vi "Canwrite_jetson.vi"(10 "클러스터":T1={"L_velocity"=0, "L_angle"=0.0, "L_Peak start"=10.0, "L_Release start"=36.0, "R_velocity"=0, "R_angle"=0.0, "R_Peak start"=10.0, "R_Release start"=36.0}) -> (2 "배열":T2(array[cluster]))   [LabVIEW 2019]
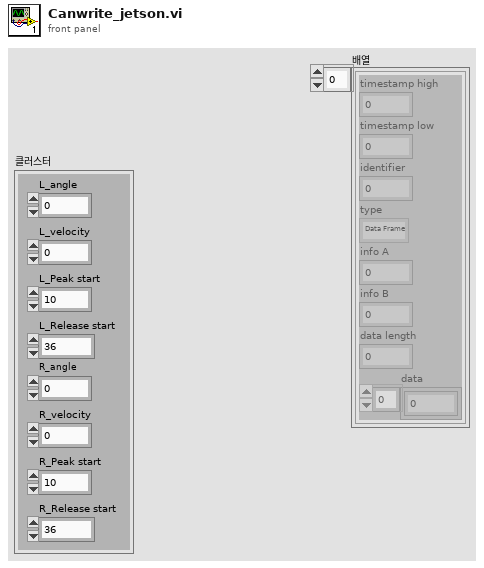
[diagram p1: front panel]
types:
  T1 = cluster{"L_velocity":u32, "L_angle":sgl, "L_Peak start":sgl, "L_Release start":sgl, "R_velocity":u32, "R_angle":sgl, "R_Peak start":sgl, "R_Release start":sgl}
  T2 = cluster{"timestamp high":u32, "timestamp low":u32, "identifier":u32, "type":enum8{"Data Frame", "Remote Frame", "(reserved)", "(reserved) ", "(reserved)  ", "(reserved)   ", "Bus Error", "Transceiver Fault"}, "info A":u8, "info B":u8, "data length":u8, "data":u8[]}[]
  T3 = enum8{"Data Frame", "Remote Frame", "(reserved)", "(reserved) ", "(reserved)  ", "(reserved)   ", "Bus Error", "Transceiver Fault"}
  T4 = cluster{"timestamp high":u32, "timestamp low":u32, "identifier":u32, "type":enum8{"Data Frame", "Remote Frame", "(reserved)", "(reserved) ", "(reserved)  ", "(reserved)   ", "Bus Error", "Transceiver Fault"}, "info A":u8, "info B":u8, "data length":u8, "data":u8[]}
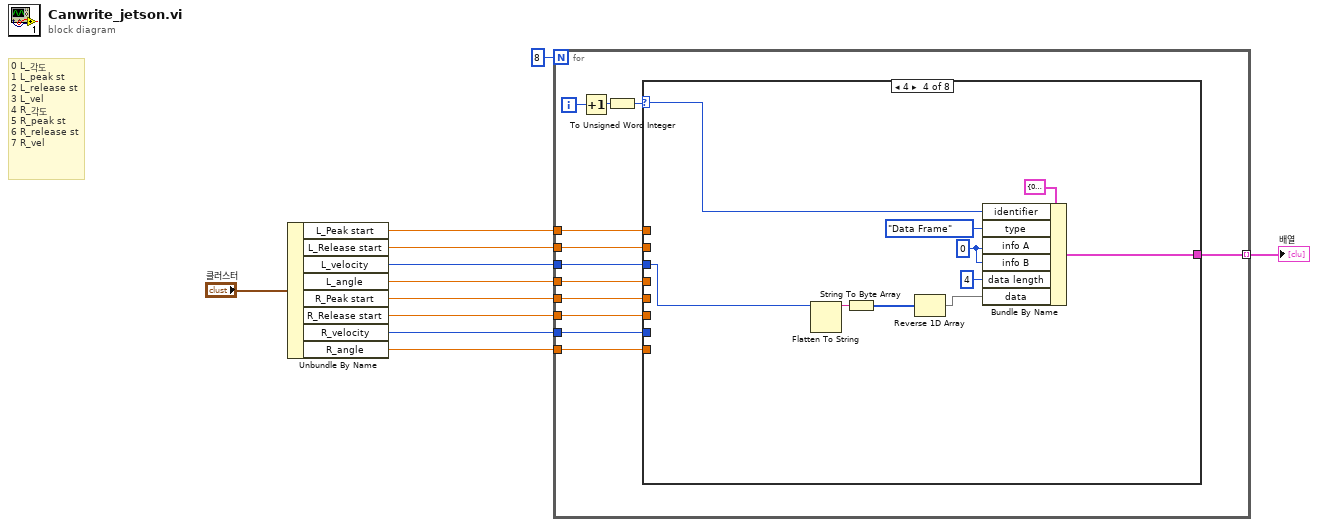
[diagram p0: block diagram]
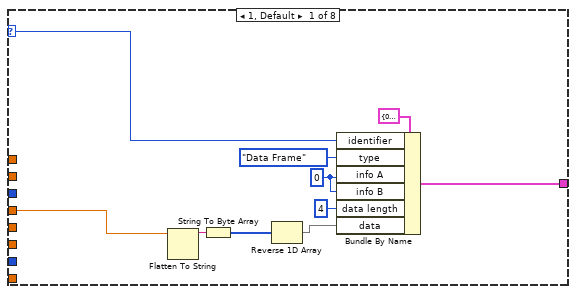
[diagram p2: hidden frame]
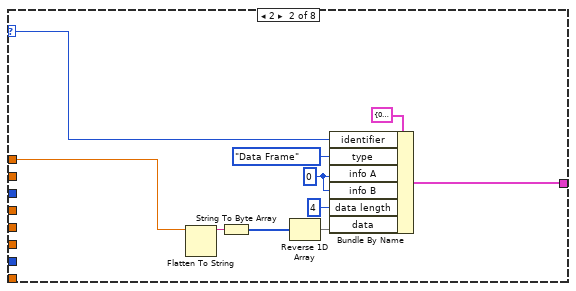
[diagram p3: hidden frame]
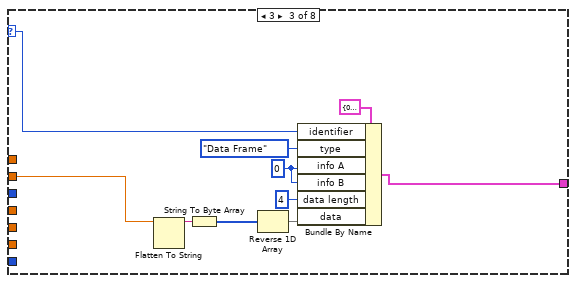
[diagram p4: hidden frame]
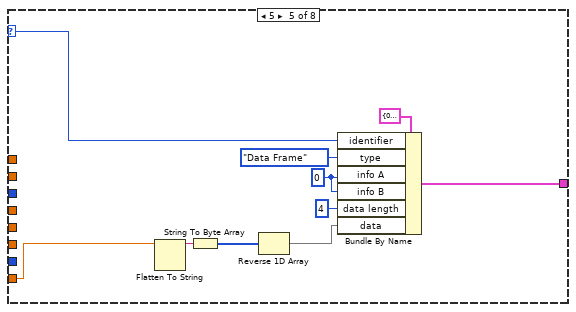
[diagram p5: hidden frame]
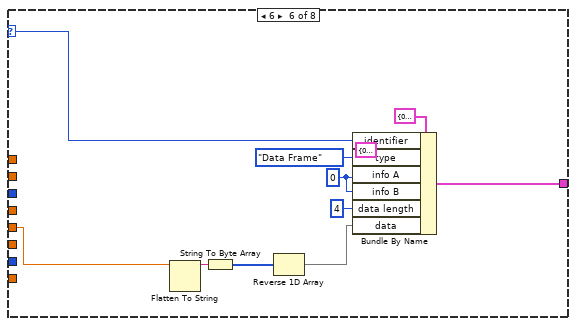
[diagram p6: hidden frame]
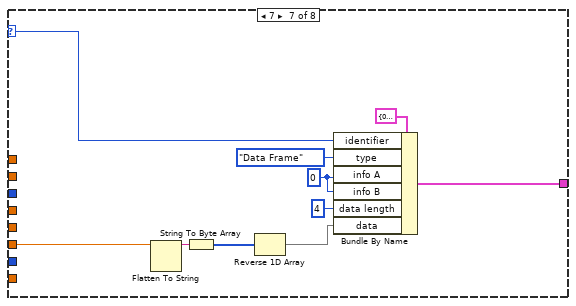
[diagram p7: hidden frame]
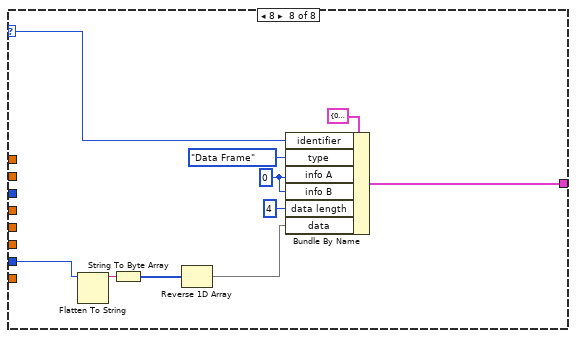
[diagram p8: hidden frame]
diagram:
  # "0 L_각도\n1 L_peak st\n2 L_release st\n3 L_vel\n4 R_각도\n5 R_peak st\n6 R_release st\n7 R_vel"
  n1 = Unbundle By Name("클러스터") -> ("L_Peak start"=w8:sgl, "L_Release start"=w6:sgl, "L_velocity"=w7:u32, "L_angle"=w5:sgl, "R_Peak start"=w4:sgl, "R_Release start"=w3:sgl, "R_velocity"=w2:u32, "R_angle"=w1:sgl)
  n2 = for {
    N: 8 -> [_]
    tunnel: w8 -> [w23]
    tunnel: w6 -> [w22]
    tunnel: w7 -> [w20]
    tunnel: [w21] -> w10 mode=indexing
    tunnel: w5 -> [w16]
    tunnel: w4 -> [w15]
    tunnel: w3 -> [w14]
    tunnel: w2 -> [w13]
    tunnel: w1 -> [w12]
    i -> [w19]
    n3 = Increment(x=w19) -> (x+1=w18:i32)
    n4 = To Unsigned Word Integer(number=w18) -> (unsigned 16bit integer=w17:u16)
    n5 = case shown="4" w17 {
      selector: w17 -> [w25 w39 w45 w59 w69 w79 w89 w99]
      tunnel: w23 -> [_ w34 _ _ _ _ _ _]
      tunnel: w22 -> [_ _ w44 _ _ _ _ _]
      tunnel: [w29 w38 w46 w58 w68 w78 w88 w98] -> w21
      tunnel: w20 -> [_ _ _ w54 _ _ _ _]
      tunnel: w16 -> [w24 _ _ _ _ _ _ _]
      tunnel: w15 -> [_ _ _ _ _ w74 _ _]
      tunnel: w14 -> [_ _ _ _ _ _ w84 _]
      tunnel: w13 -> [_ _ _ _ _ _ _ w94]
      tunnel: w12 -> [_ _ _ _ w64 _ _ _]
      frame 1, Default {
        w31 = u8 0 ("info A")
        n6 = Flatten To String(anything=w24) -> (data string=w28:string)  [unwired: 3 in, 2 out]
        n7 = String To Byte Array(string=w28) -> (unsigned byte array=w27:u8[])
        n8 = Reverse 1D Array(array=w27) -> (reversed array=w26:u8[])
        n9 = Bundle By Name(cluster=T4 {"timestamp high"=0, "timestamp low"=0, "identifier"=0, "type"=enum."Data Frame", "info A"=0, "info B"=0, "data length"=0, "data"=[0, 0, 0, 0, 0, 0, 0, 0]} ("출력 클러스터"), "identifier"=w25, "type"=T3."Data Frame", "info A"=w31, "info B"=w31, "data length"=u8 4, "data"=w26) -> (w29:T4)
      }
      frame 2 {
        w41 = u8 0 ("info A")
        n10 = Flatten To String(anything=w34) -> (data string=w37:string)  [unwired: 3 in, 2 out]
        n11 = String To Byte Array(string=w37) -> (unsigned byte array=w36:u8[])
        n12 = Reverse 1D Array(array=w36) -> (reversed array=w35:u8[])
        n13 = Bundle By Name(cluster=T4 {"timestamp high"=0, "timestamp low"=0, "identifier"=0, "type"=enum."Data Frame", "info A"=0, "info B"=0, "data length"=0, "data"=[0, 0, 0, 0, 0, 0, 0, 0]} ("출력 클러스터"), "identifier"=w39, "type"=T3."Data Frame", "info A"=w41, "info B"=w41, "data length"=u8 4, "data"=w35) -> (w38:T4)
      }
      frame 3 {
        w51 = u8 0 ("info A")
        n14 = Flatten To String(anything=w44) -> (data string=w49:string)  [unwired: 3 in, 2 out]
        n15 = String To Byte Array(string=w49) -> (unsigned byte array=w48:u8[])
        n16 = Reverse 1D Array(array=w48) -> (reversed array=w47:u8[])
        n17 = Bundle By Name(cluster=T4 {"timestamp high"=0, "timestamp low"=0, "identifier"=0, "type"=enum."Data Frame", "info A"=0, "info B"=0, "data length"=0, "data"=[0, 0, 0, 0, 0, 0, 0, 0]} ("출력 클러스터"), "identifier"=w45, "type"=T3."Data Frame", "info A"=w51, "info B"=w51, "data length"=u8 4, "data"=w47) -> (w46:T4)
      }
      frame 4 {
        w61 = u8 0 ("info A")
        n18 = Flatten To String(anything=w54) -> (data string=w57:string)  [unwired: 3 in, 2 out]
        n19 = String To Byte Array(string=w57) -> (unsigned byte array=w56:u8[])
        n20 = Reverse 1D Array(array=w56) -> (reversed array=w55:u8[])
        n21 = Bundle By Name(cluster=T4 {"timestamp high"=0, "timestamp low"=0, "identifier"=0, "type"=enum."Data Frame", "info A"=0, "info B"=0, "data length"=0, "data"=[0, 0, 0, 0, 0, 0, 0, 0]} ("출력 클러스터"), "identifier"=w59, "type"=T3."Data Frame", "info A"=w61, "info B"=w61, "data length"=u8 4, "data"=w55) -> (w58:T4)
      }
      frame 5 {
        w71 = u8 0 ("info A")
        n22 = Flatten To String(anything=w64) -> (data string=w67:string)  [unwired: 3 in, 2 out]
        n23 = String To Byte Array(string=w67) -> (unsigned byte array=w66:u8[])
        n24 = Reverse 1D Array(array=w66) -> (reversed array=w65:u8[])
        n25 = Bundle By Name(cluster=T4 {"timestamp high"=0, "timestamp low"=0, "identifier"=0, "type"=enum."Data Frame", "info A"=0, "info B"=0, "data length"=0, "data"=[0, 0, 0, 0, 0, 0, 0, 0]} ("출력 클러스터"), "identifier"=w69, "type"=T3."Data Frame", "info A"=w71, "info B"=w71, "data length"=u8 4, "data"=w65) -> (w68:T4)
      }
      frame 6 {
        (unwired) T4 {"timestamp high"=0, "timestamp low"=0, "identifier"=0, "type"=enum."Data Frame", "info A"=0, "info B"=0, "data length"=0, "data"=[0, 0, 0, 0, 0, 0, 0, 0]} ("출력 클러스터")
        w81 = u8 0 ("info A")
        n26 = Flatten To String(anything=w74) -> (data string=w77:string)  [unwired: 3 in, 2 out]
        n27 = String To Byte Array(string=w77) -> (unsigned byte array=w76:u8[])
        n28 = Reverse 1D Array(array=w76) -> (reversed array=w75:u8[])
        n29 = Bundle By Name(cluster=T4 {"timestamp high"=0, "timestamp low"=0, "identifier"=0, "type"=enum."Data Frame", "info A"=0, "info B"=0, "data length"=0, "data"=[0, 0, 0, 0, 0, 0, 0, 0]} ("출력 클러스터"), "identifier"=w79, "type"=T3."Data Frame", "info A"=w81, "info B"=w81, "data length"=u8 4, "data"=w75) -> (w78:T4)
      }
      frame 7 {
        w91 = u8 0 ("info A")
        n30 = Flatten To String(anything=w84) -> (data string=w87:string)  [unwired: 3 in, 2 out]
        n31 = String To Byte Array(string=w87) -> (unsigned byte array=w86:u8[])
        n32 = Reverse 1D Array(array=w86) -> (reversed array=w85:u8[])
        n33 = Bundle By Name(cluster=T4 {"timestamp high"=0, "timestamp low"=0, "identifier"=0, "type"=enum."Data Frame", "info A"=0, "info B"=0, "data length"=0, "data"=[0, 0, 0, 0, 0, 0, 0, 0]} ("출력 클러스터"), "identifier"=w89, "type"=T3."Data Frame", "info A"=w91, "info B"=w91, "data length"=u8 4, "data"=w85) -> (w88:T4)
      }
      frame 8 {
        w101 = u8 0 ("info A")
        n34 = Flatten To String(anything=w94) -> (data string=w97:string)  [unwired: 3 in, 2 out]
        n35 = String To Byte Array(string=w97) -> (unsigned byte array=w96:u8[])
        n36 = Reverse 1D Array(array=w96) -> (reversed array=w95:u8[])
        n37 = Bundle By Name(cluster=T4 {"timestamp high"=0, "timestamp low"=0, "identifier"=0, "type"=enum."Data Frame", "info A"=0, "info B"=0, "data length"=0, "data"=[0, 0, 0, 0, 0, 0, 0, 0]} ("출력 클러스터"), "identifier"=w99, "type"=T3."Data Frame", "info A"=w101, "info B"=w101, "data length"=u8 4, "data"=w95) -> (w98:T4)
      }
    }
  }
  "배열" <- w10
